vi "Write Task Name.vi"(8 "error in (no error)":errorcluster, 10 "Task Name":string, 11 "Task Ancestor in":refnum<class "Task Ancestor.lvclass">) -> (0 "error out":errorcluster, 3 "Task Ancestor out":refnum<class "Task Ancestor.lvclass">)   [LabVIEW 2024, in "Task Ancestor.lvclass"]
uses:
  Task Ancestor.lvclass
  Task Ancestor.lvclass/Task Ancestor.ctl
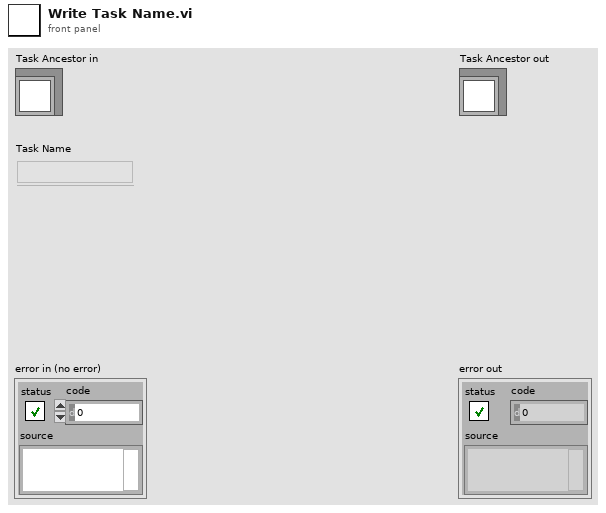
[diagram p1: front panel]
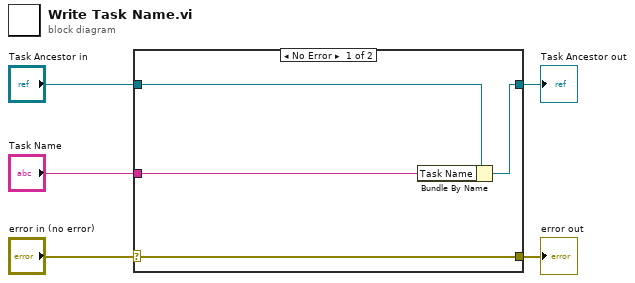
[diagram p0: block diagram]
diagram:
  n1 = case shown="No Error" "error in (no error)" {
    selector: "error in (no error)" -> [w9 w10]
    tunnel: [w9 w10] -> w4
    tunnel: [w7 w11] -> w2
    tunnel: "Task Ancestor in" -> [w8 w11]
    tunnel: "Task Name" -> [w6 _]
    frame No Error {
      n2 = Bundle By Name(cluster=w8, "Task Name"=w6) -> (w7:refnum<class "Task Ancestor.lvclass">)
    }
    frame Error {
    }
  }
  "error out" <- w4
  "Task Ancestor out" <- w2
